vi "ReadSerialAsync.vi"(5 "IDmap":map{string, T3}(c390), 7 "CmdMap":map{string, T2}(c390), 10 "input Str":string) -> (1 "Status":string, 2 "ID":string, 3 "Category":string, 4 "PrinterCmdStatus":T1)   [LabVIEW 2022 SP3, in "GIS Printer.lvclass"]
uses:
  GIS Printer/GIS Printer.lvclass
  GIS Printer/Typedefs/PrinterCommand--Cluster.ctl
  GIS Printer/Typedefs/PrinterCmdStatus--Enum.ctl
  GIS Printer/Typedefs/PrinterResponse--Cluster.ctl
  <vilib>/Utility/miscctls.llb/LVMapReplaceAction.ctl
panel:
  out "CmdMapout":map{string, T2}(c390)
  out "IDmap out":map{string, T3}(c390)
  out "error out":errorcluster
  in  "error in":errorcluster
  # "I,[ID],RTP,1"
  # "C,[ID],0"
  # "A,[ID],P,C,P,\"Print Manager,Print Line Manager,PMB-KM,PrintGoSource\",\"TTL\""
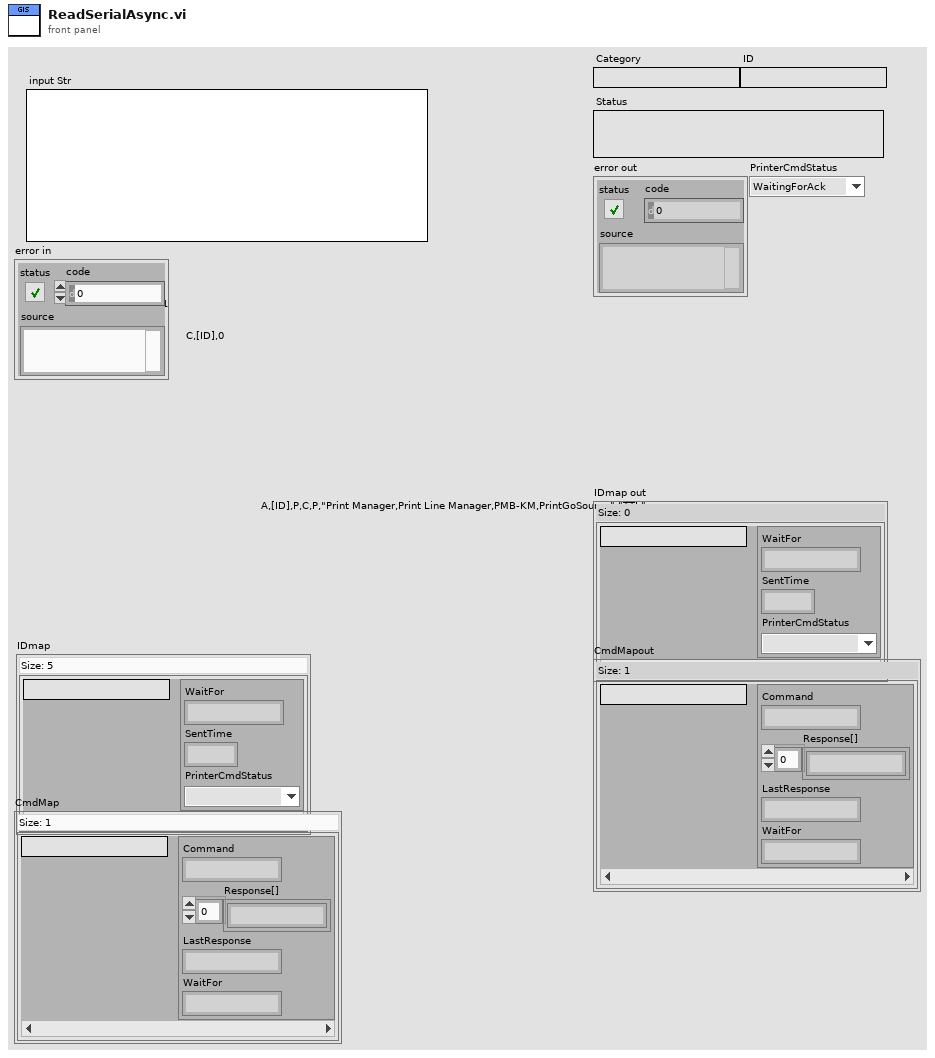
[diagram p1: front panel]
types:
  T1 = typedef "GIS Printer.lvclass/PrinterCmdStatus--Enum.ctl" = enum16{"WaitingForAck", "Executing", "Executing Standby", "Completed", "Error"}
  T2 = typedef "GIS Printer.lvclass/PrinterResponse--Cluster.ctl" = cluster{"Command":string, "Response[]":string[], "LastResponse":string, "WaitFor":string}
  T3 = typedef "GIS Printer.lvclass/PrinterCommand--Cluster.ctl" = cluster{"WaitFor":string, "SentTime":dbl, "PrinterCmdStatus":T1}
  T4 = typedef "LVMapReplaceAction.ctl" = enum32{"Modify Entry only if found", "Add or Modify Entry", "Delete Entry"}
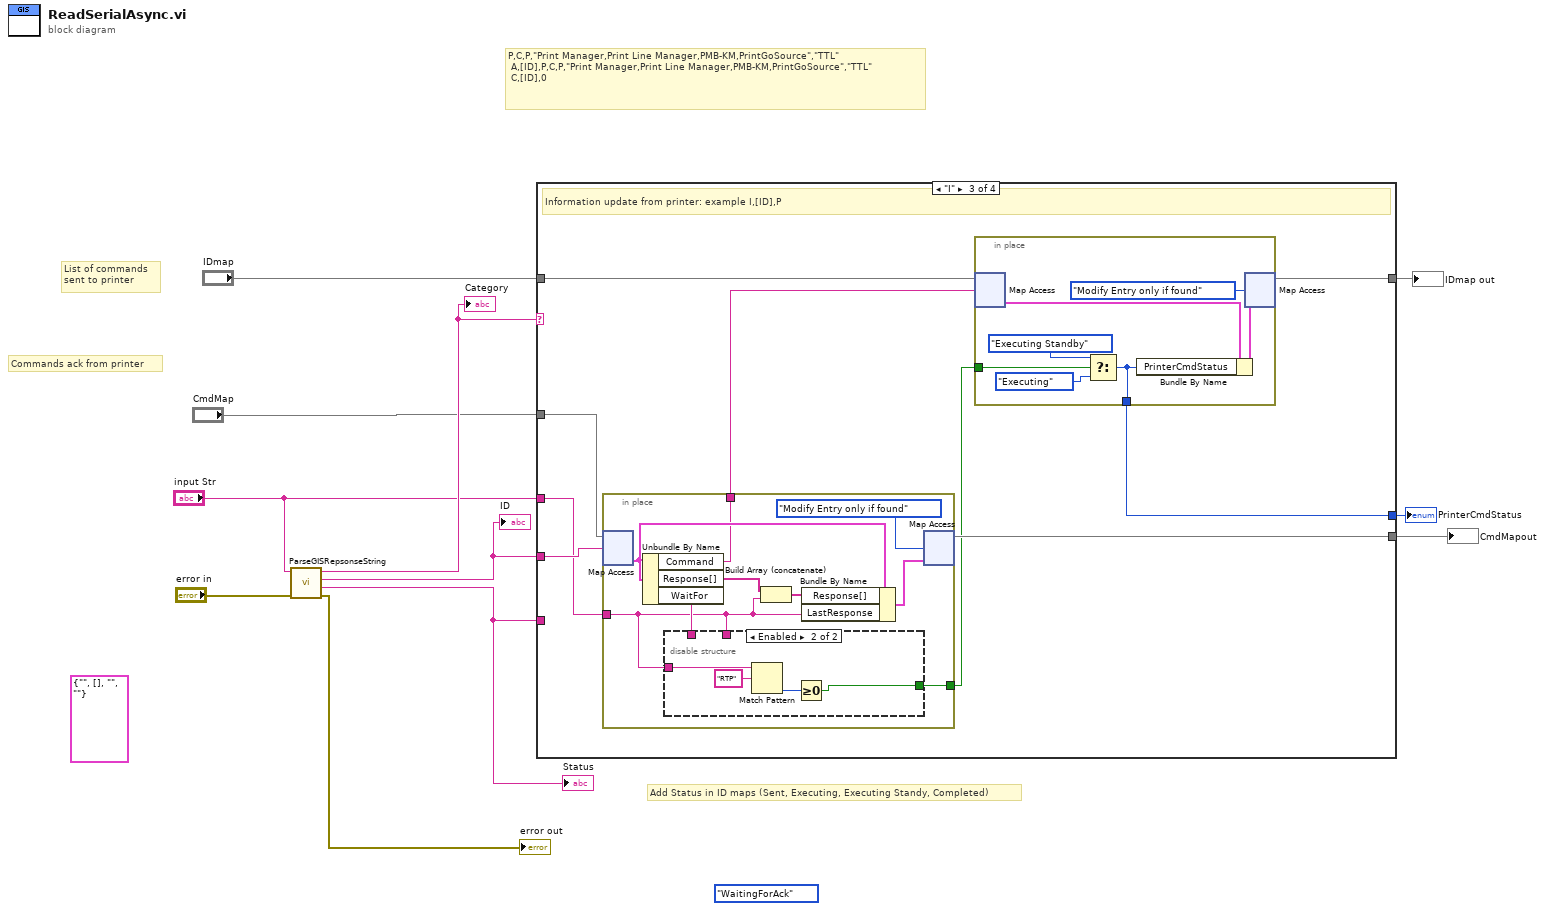
[diagram p0: block diagram]
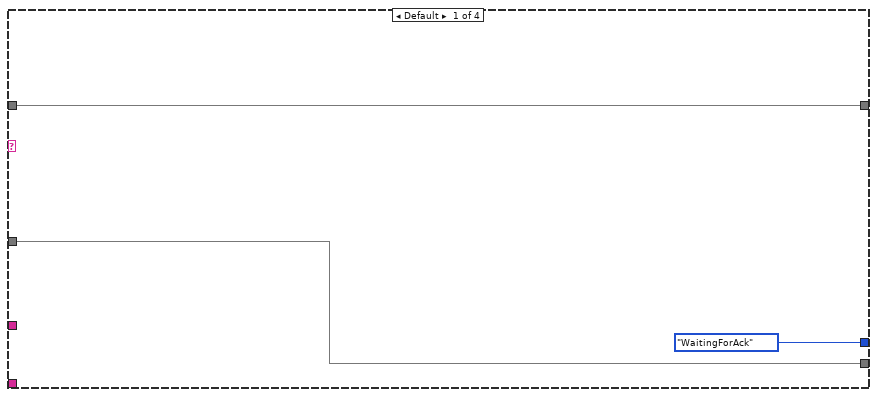
[diagram p2: hidden frame]
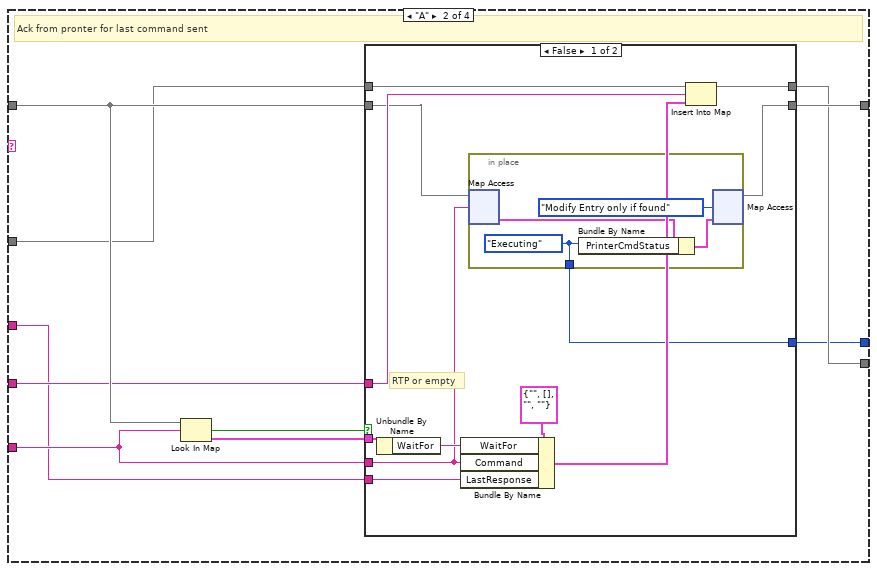
[diagram p3: hidden frame]
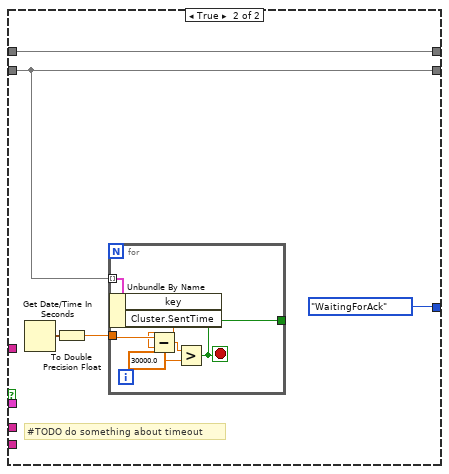
[diagram p4: hidden frame]
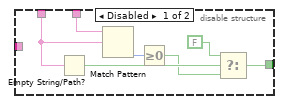
[diagram p5: hidden frame]
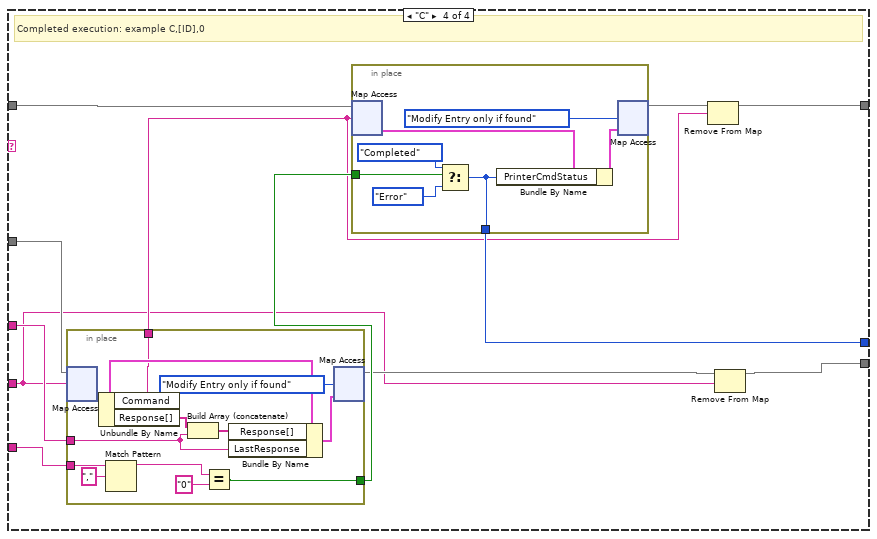
[diagram p6: hidden frame]
diagram:
  (unwired) PrinterCmdStatus--Enum."WaitingForAck" ("PrinterCmdStatus")
  (unwired) T2 {"Command"="", "Response[]"=[], "LastResponse"="", "WaitFor"=""}
  # "Commands ack from printer"
  # "List of commands\nsent to printer"
  # "Add Status in ID maps (Sent, Executing, Executing Standy, Completed)"
  # "P,C,P,\"Print Manager,Print Line Manager,PMB-KM,PrintGoSource\",\"TTL\"\t\n\tA,[ID],P,C,P,\"Print Manager,Print Line Manager,PMB-KM,PrintGoSource\",\"TTL\"\n\tC,[ID],0"
  n1 = call "ParseGISRepsonseString.vi"("error in (no error)"="error in", "Response In"="input Str") -> ("error out"=→"error out":errorcluster, "Status"=w9:string, "ID"=w10:string, "Category"=w11:string)  [unwired: 6 in]
  "Category" <- w11
  "ID" <- w10
  "Status" <- w9
  n2 = case shown="\"I\"" w11 {
    tunnel: w10 -> [_ w20 w59 w88]
    tunnel: w9 -> [_ w21 _ w94]
    tunnel: "IDmap" -> [w13 w23 w55 w97]
    tunnel: [w13 w24 w56 w92] -> w3
    tunnel: "CmdMap" -> [w14 w19 w60 w99]
    tunnel: [w14 w18 w57 w89] -> w2
    tunnel: "input Str" -> [_ w17 w58 w98]
    tunnel: [PrinterCmdStatus--Enum."WaitingForAck" ("PrinterCmdStatus") w15 w53 w95] -> w1
    frame Default {
    }
    frame "A" {
      # "Ack from pronter for last command sent"
      n3 = Look In Map(map=w23, key=w21) -> (key not found?=w22:bool, value=w16:T3)  [unwired: 1 in]
      n4 = case shown="False" w22 {
        tunnel: w23 -> [w28 w45]
        tunnel: [w27 w45] -> w24
        tunnel: w21 -> [w26 _]
        tunnel: w20 -> [w34 _]
        tunnel: w19 -> [w36 w42]
        tunnel: [w33 w42] -> w18
        tunnel: w17 -> [w32 _]
        tunnel: w16 -> [w30 _]
        tunnel: [w25 PrinterCmdStatus--Enum."WaitingForAck" ("PrinterCmdStatus")] -> w15
        frame False {
          # "RTP or empty"
          n5 = Unbundle By Name(w30) -> ("WaitFor"=w29:string)
          n6 = Bundle By Name(cluster=T2 {"Command"="", "Response[]"=[], "LastResponse"="", "WaitFor"=""} ("value"), "WaitFor"=w29, "Command"=w26, "LastResponse"=w32) -> (w31:T2)
          n7 = in-place {
            in-place-border: [w37] -> w25
            w37 = PrinterCmdStatus--Enum."Executing" ("PrinterCmdStatus")
            n8 = in-place-map #1(w28, w26) -> (w40:T3)  [unwired: 1 in, 1 out]
            n9 = Bundle By Name(cluster=w40, "PrinterCmdStatus"=w37) -> (w38:T3)
            n10 = in-place-map #1(w38, LVMapReplaceAction."Modify Entry only if found" ("action")) -> (w27:map{string, T3})  [unwired: 2 out]
          }
          n11 = Insert Into Map(map in=w36, key=w34, value=w31) -> (map out=w33:map{string, T2})  [unwired: 2 out]
        }
        frame True {
          # "#TODO do something about timeout"
          n12 = Get Date/Time In Seconds() -> (seconds since 1Jan1904=w44:timestamp)
          n13 = To Double Precision Float(number=w44) -> (double precision float=w43:dbl)
          n14 = for {
            tunnel: w45 -> [w51] mode=indexing
            tunnel: w43 -> [w49]
            tunnel: [w46] -> _
            stop <- w46 stop-if-true
            n15 = Unbundle By Name(w51) -> ("Cluster.SentTime"=w48:dbl)  [unwired: 1 out]
            n16 = Subtract(x=w49, y=w48) -> (x-y=w50:dbl)
            n17 = Greater?(x=w50, y=30000.0) -> (0:w46:bool)
          }
        }
      }
    }
    frame "I" {
      # "Information update from printer: example I,[ID],P"
      n18 = in-place {
        in-place-border: w58 -> [w68]
        in-place-border: [w70] -> w52
        in-place-border: [w69] -> w54
        n19 = in-place-map #2(w60, w59) -> (w76:T2)  [unwired: 1 in, 1 out]
        n20 = Unbundle By Name(w76) -> ("Command"=w69:string, "Response[]"=w75:string[], "WaitFor"=w71:string)
        n21 = disable-structure shown="Enabled" {
          disable-tunnel: w68 -> [w83 _]
          disable-tunnel: w71 -> [w81 _]
          disable-tunnel: [w77 w84] -> w70
          disable-tunnel: w68 -> [_ w87]
          frame Disabled {
            n22 = Empty String/Path?(string/path=w81) -> (empty?=w80:bool)
            n23 = Match Pattern(string=w83, regular expression=w81) -> (offset past match=w82:i32)  [unwired: 1 in, 3 out]
            n24 = Greater Or Equal To 0?(x=w82) -> (x >= 0?=w78:bool)
            n25 = Select(t=FALSE, s=w80, f=w78) -> (s? t:f=w77:bool)
          }
          frame Enabled {
            n26 = Match Pattern(string=w87, regular expression="RTP") -> (offset past match=w85:i32)  [unwired: 1 in, 3 out]
            n27 = Greater Or Equal To 0?(x=w85) -> (x >= 0?=w84:bool)
          }
        }
        n28 = Build Array (concatenate)(w75, w68) -> (w74:string[])
        n29 = Bundle By Name(cluster=w76, "Response[]"=w74, "LastResponse"=w68) -> (w73:T2)
        n30 = in-place-map #2(w73, LVMapReplaceAction."Modify Entry only if found" ("action")) -> (w57:map{string, T2})  [unwired: 2 out]
      }
      n31 = in-place {
        in-place-border: [w61] -> w53
        in-place-border: w52 -> [w64]
        n32 = in-place-map #3(w55, w54) -> (w67:T3)  [unwired: 1 in, 1 out]
        n33 = Select(t=PrinterCmdStatus--Enum."Executing Standby" ("PrinterCmdStatus"), s=w64, f=PrinterCmdStatus--Enum."Executing") -> (s? t:f=w61:T1)
        n34 = Bundle By Name(cluster=w67, "PrinterCmdStatus"=w61) -> (w65:T3)
        n35 = in-place-map #3(w65, LVMapReplaceAction."Modify Entry only if found" ("action")) -> (w56:map{string, T3})  [unwired: 2 out]
      }
    }
    frame "C" {
      # "Completed execution: example C,[ID],0"
      n36 = in-place {
        in-place-border: w98 -> [w112]
        in-place-border: [w113] -> w91
        in-place-border: [w110] -> w96
        in-place-border: w94 -> [w109]
        n37 = in-place-map #4(w99, w88) -> (w114:T2)  [unwired: 1 in, 1 out]
        n38 = Unbundle By Name(w114) -> ("Command"=w113:string, "Response[]"=w118:string[])
        n39 = Match Pattern(string=w109, regular expression=",") -> (before substring=w107:string)  [unwired: 1 in, 3 out]
        n40 = Build Array (concatenate)(w118, w112) -> (w117:string[])
        n41 = Equal?(x=w107, y="0") -> (x = y?=w110:bool)
        n42 = Bundle By Name(cluster=w114, "Response[]"=w117, "LastResponse"=w112) -> (w116:T2)
        n43 = in-place-map #4(w116, LVMapReplaceAction."Modify Entry only if found" ("action")) -> (w90:map{string, T2})  [unwired: 2 out]
      }
      n44 = in-place {
        in-place-border: w96 -> [w104]
        in-place-border: [w100] -> w95
        n45 = in-place-map #5(w97, w91) -> (w106:T3)  [unwired: 1 in, 1 out]
        n46 = Select(t=PrinterCmdStatus--Enum."Completed" ("PrinterCmdStatus"), s=w104, f=PrinterCmdStatus--Enum."Error" ("PrinterCmdStatus")) -> (s? t:f=w100:T1)
        n47 = Bundle By Name(cluster=w106, "PrinterCmdStatus"=w100) -> (w101:T3)
        n48 = in-place-map #5(w101, LVMapReplaceAction."Modify Entry only if found" ("action")) -> (w93:map{string, T3})  [unwired: 2 out]
      }
      n49 = Remove From Map(10:w91, 11:w93) -> (3:w92:map{string, T3})  [unwired: 2 out]
      n50 = Remove From Map(10:w88, 11:w90) -> (3:w89:map{string, T2})  [unwired: 2 out]
    }
  }
  "IDmap out" <- w3
  "CmdMapout" <- w2
  "PrinterCmdStatus" <- w1
